vi "Convert Time(String) To Num.vi"(11 "ExcuseTime(\"\")":string) -> (2 "Time2":i32, 3 "Time1":i32)   [LabVIEW 2015, in "Admin_Actor.lvlib" / "ExcuseNotesHandler.lvclass"]
uses:
  ExcuseNotesHandler.lvclass
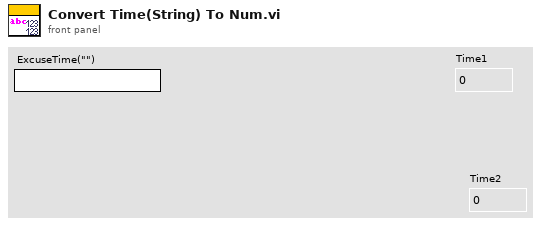
[diagram p1: front panel]
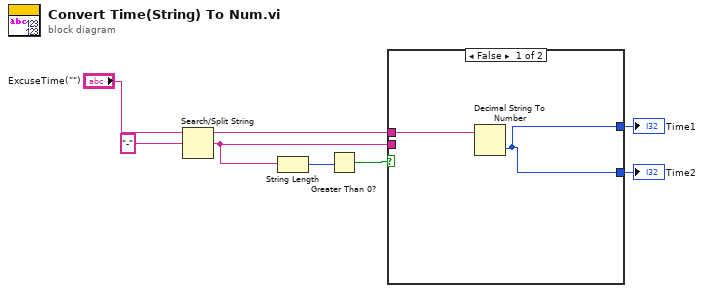
[diagram p0: block diagram]
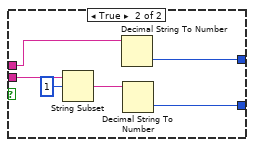
[diagram p2: hidden frame]
diagram:
  n1 = Search/Split String(string="ExcuseTime(\"\")", search string/char (-)="-") -> (substring before match=w5:string, match + rest of string=w4:string)  [unwired: 1 in, 1 out]
  n2 = String Length(string=w4) -> (length=w6:i32)
  n3 = Greater Than 0?(x=w6) -> (x > 0?=w1:bool)
  n4 = case shown="False" w1 {
    tunnel: w5 -> [w10 w12]
    tunnel: w4 -> [_ w16]
    tunnel: [w9 w13] -> w2
    tunnel: [w9 w11] -> w3
    frame False {
      n5 = Decimal String To Number(string=w10) -> (number=w9:i32)  [unwired: 2 in, 1 out]
    }
    frame True {
      n6 = String Subset(string=w16, offset (0)=1) -> (substring=w14:string)  [unwired: 1 in]
      n7 = Decimal String To Number(string=w12) -> (number=w11:i32)  [unwired: 2 in, 1 out]
      n8 = Decimal String To Number(string=w14) -> (number=w13:i32)  [unwired: 2 in, 1 out]
    }
  }
  "Time1" <- w3
  "Time2" <- w2
